vi "Extract MultiSourceFrame Data.vi"(6 "Data Type Enabled?":bool, 8 "error in (no error)":errorcluster, 9 "MultiSourceFrame Reference in":refnum<k24>, 10 "Frame Data Type":i32, 11 "Frame Data in":variant) -> (0 "error out":errorcluster, 2 "Boolean":bool, 3 "Frame Data out":variant)   [LabVIEW 2014, in "LVH-KinectOne.lvlib"]
uses:
  LVH-KinectOne.lvlib
  Microsoft.Kinect
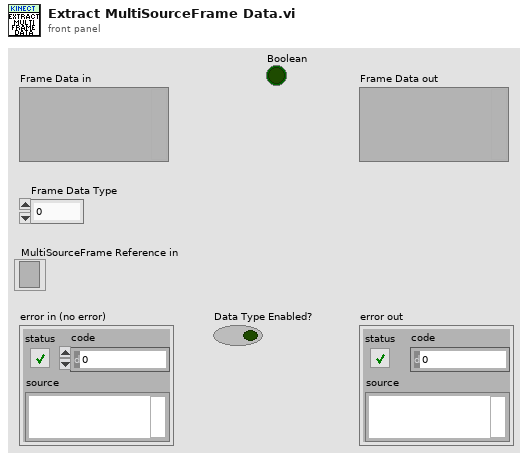
[diagram p1: front panel]
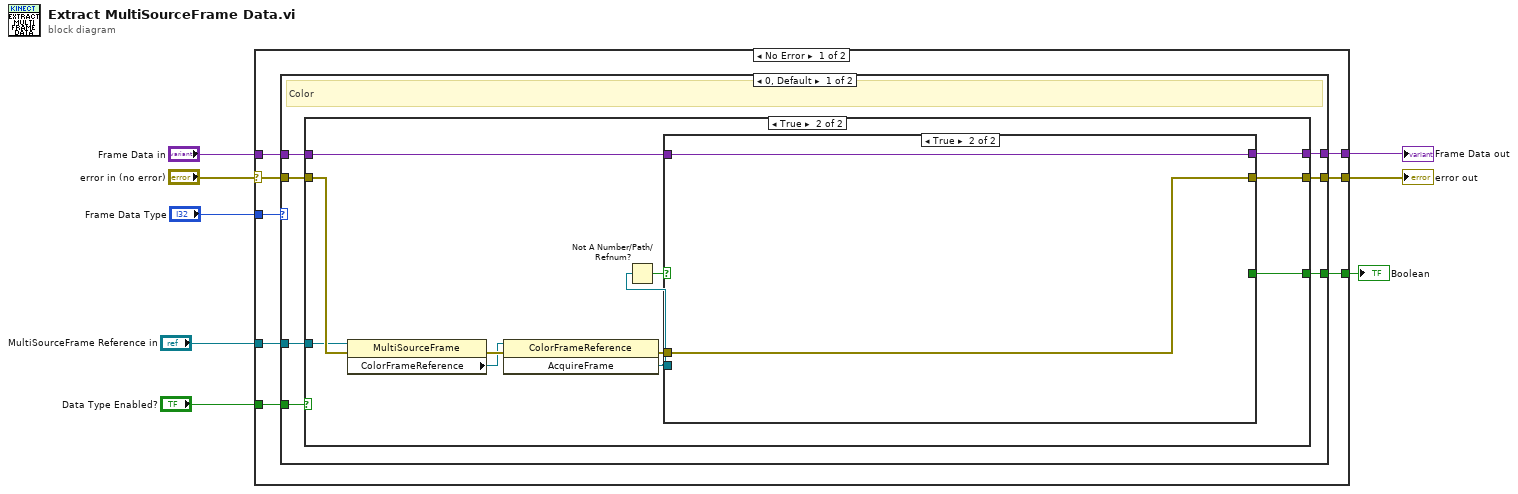
[diagram p0: block diagram]
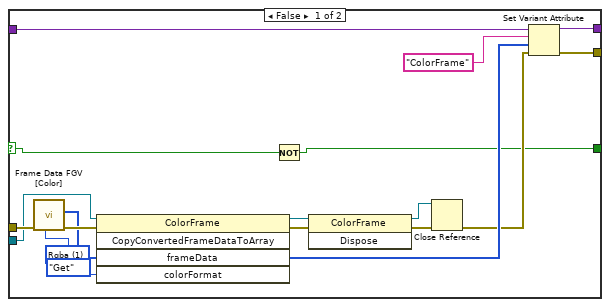
[diagram p3: hidden frame]
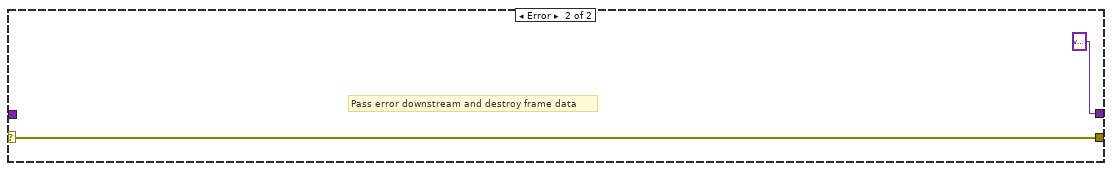
[diagram p5: hidden frame]
diagram:
  n1 = case shown="No Error" "error in (no error)" {
    selector: "error in (no error)" -> [w11 w60]
    tunnel: [w16 variant] -> w2
    tunnel: [w15 w60] -> w3
    tunnel: "Frame Data in" -> [w12 _]
    tunnel: "Frame Data Type" -> [w14 _]
    tunnel: "Data Type Enabled?" -> [w13 _]
    tunnel: "MultiSourceFrame Reference in" -> [w10 _]
    tunnel: [w9 _] -> w1
    frame No Error {
      n2 = case shown="0, Default" w14 {
        tunnel: [w23 w58] -> w16
        tunnel: [w22 w57] -> w15
        tunnel: w13 -> [w21 _]
        tunnel: w12 -> [w20 w58]
        tunnel: w11 -> [w19 w57]
        tunnel: w10 -> [w18 _]
        tunnel: [w17 _] -> w9
        frame 0, Default {
          # "Color"
          n3 = case shown="True" w21 {
            tunnel: [w25 w36] -> w23
            tunnel: [w24 w35] -> w22
            tunnel: w20 -> [w25 w33]
            tunnel: w19 -> [w24 w34]
            tunnel: w18 -> [_ w31]
            tunnel: [_ w26] -> w17
            frame False {
            }
            frame True {
              n4 = property class="MultiSourceFrame"(reference=w31, error in=w34) -> (error out=w32:errorcluster, "ColorFrameReference"=w30:refnum<k24>)  [unwired: 1 out]
              n5 = invoke class="ColorFrameReference" method="AcquireFrame"(reference=w30, error in=w32) -> (error out=w29:errorcluster, "AcquireFrame"=w27:refnum<k24>)  [unwired: 1 in, 1 out]
              n6 = Not A Number/Path/Refnum?(number/path/refnum=w27) -> (NaN/Path/Refnum?=w28:bool)
              n7 = case shown="True" w28 {
                selector: w28 -> [w38 _]
                tunnel: [w54 w55] -> w36
                tunnel: [w53 w56] -> w35
                tunnel: w33 -> [w51 w55]
                tunnel: w29 -> [w40 w56]
                tunnel: w27 -> [w39 _]
                tunnel: [w37 _] -> w26
                frame False {
                  w41 = 1 items=["None", "Rgba", "Yuv", "Bgra", "Bayer", "Yuy2"] ("colorFormat")
                  n8 = call "Frame Data FGV [Color].vi"("Command"=enum16{"Get", "Initialize"}."Get", "error in (no error)"=w40) -> ("error out"=w49:errorcluster, "Byte Array"=w43:u8[])  [unwired: 8 in]
                  n9 = invoke class="ColorFrame" method="CopyConvertedFrameDataToArray"(reference=w39, error in=w49, "frameData"=w43, "colorFormat"=w41) -> (reference out=w45:refnum<k24>, error out=w46:errorcluster, "frameData"=w50:u8[])  [unwired: 1 in, 2 out]
                  n10 = Not(x=w38) -> (.not. x?=w37:bool)
                  n11 = invoke class="ColorFrame" method="Dispose"(reference=w45, error in=w46) -> (reference out=w48:refnum<k24>, error out=w47:errorcluster)  [unwired: 1 in, 1 out]
                  n12 = Close Reference(reference=w48, error in (no error)=w47) -> (error out=w44:errorcluster)
                  n13 = Set Variant Attribute(Variant=w51, name="ColorFrame", value=w50, error in=w44) -> (Variant out=w54:variant, error out=w53:errorcluster)  [unwired: 1 out]
                }
                frame True {
                }
              }
            }
          }
        }
        frame 1 {
          # "Infrared"
        }
      }
    }
    frame Error {
      # "Pass error downstream and destroy frame data"
    }
  }
  "error out" <- w3
  "Frame Data out" <- w2
  "Boolean" <- w1
